vi "Test My Singleton Module API.vi"() -> ()   [LabVIEW 2017]
doc: "My Singleton Module API Tester.\n_____\nBased on Delacor QMH Project Template 3.1.0.34."
uses:
  My Singleton Module.lvlib
panel:
  out "LED":bool
  in  "Digital control":bool
  in  "Show Block Diagram":bool
  in  "X":dbl=1.0
  out "Reply Payload":dbl
  out "Reply Received?":bool
  in  "Stop Module":bool
  in  "Start Module":bool
  out "Do Something Count":i32
  in  "Test Do Something Else and Wait for Reply":bool
  in  "Hide Module Panel":bool
  in  "Show Module Panel":bool
  in  "Test Do Something Else":bool
  in  "Test Do Something":bool
  out "Status":string
  out "Module Running?":bool
  # "This VI tests the API for the Module."
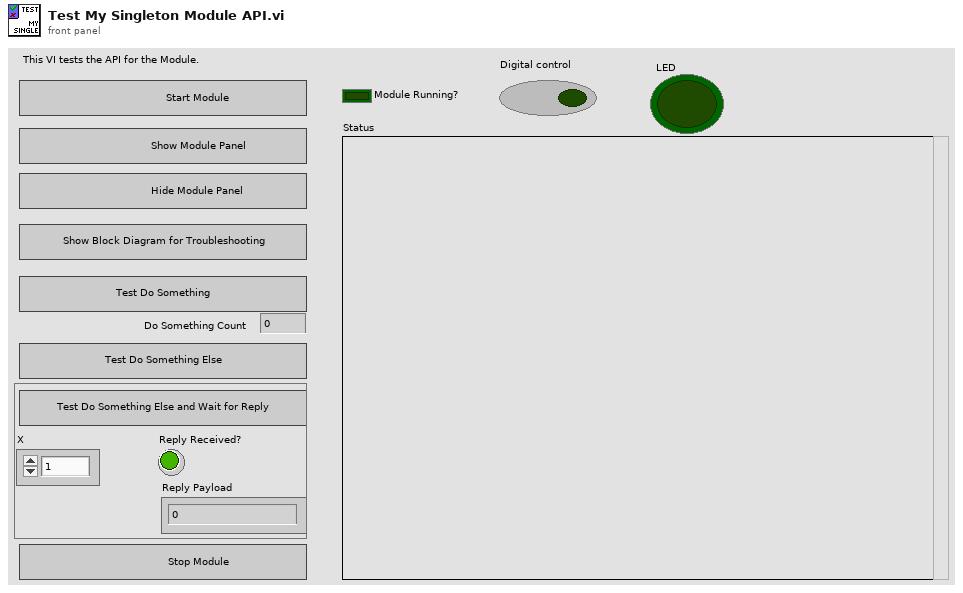
[diagram p1: front panel]
types:
  T1 = typedef "My Singleton Module.lvlib/Broadcast Events--cluster.ctl" = cluster{"Module Did Init":refnum<user-event>, "Status Updated":refnum<user-event>, "Error Reported":refnum<user-event>, "Did Something":refnum<user-event>, "Module Did Stop":refnum<user-event>, "Update Module Execution Status":refnum<user-event>}
  T2 = typedef "My Singleton Module.lvlib/Do Something Else and Wait (Reply Payload)--cluster.ctl" = cluster{"Value":dbl, "error":errorcluster}
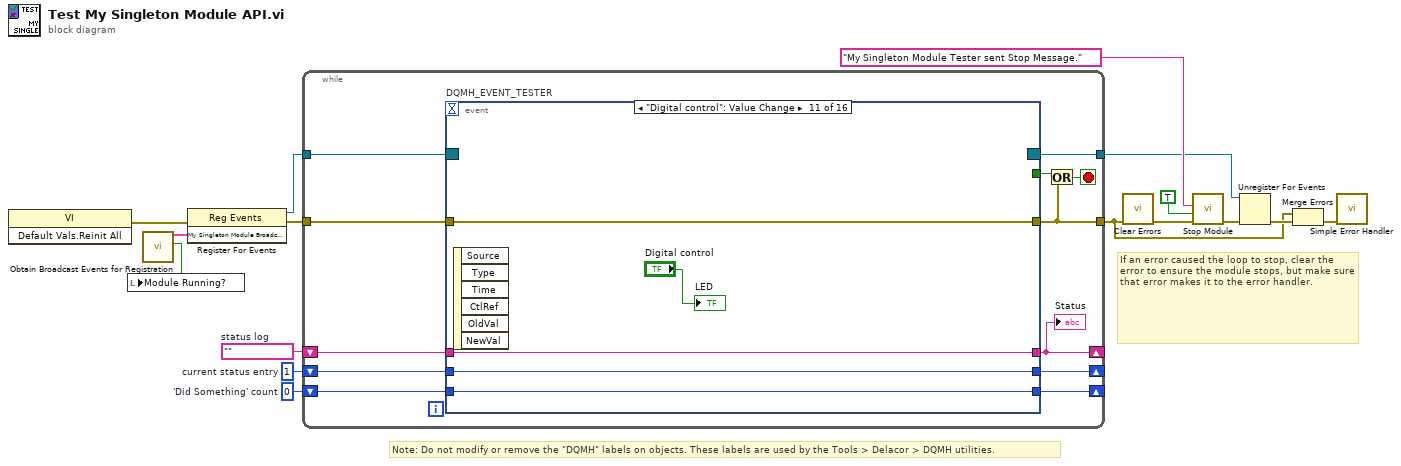
[diagram p0: block diagram]
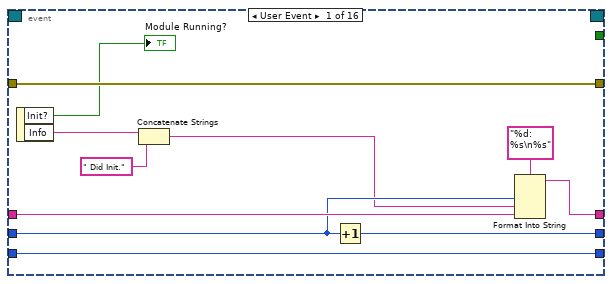
[diagram p2: hidden frame]
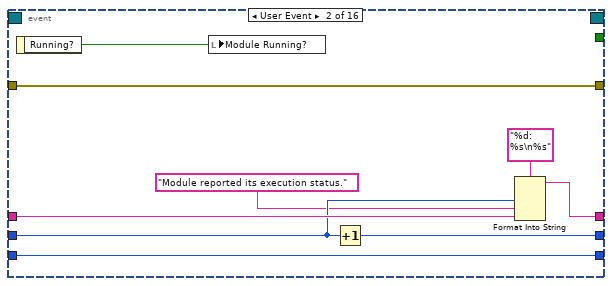
[diagram p3: hidden frame]
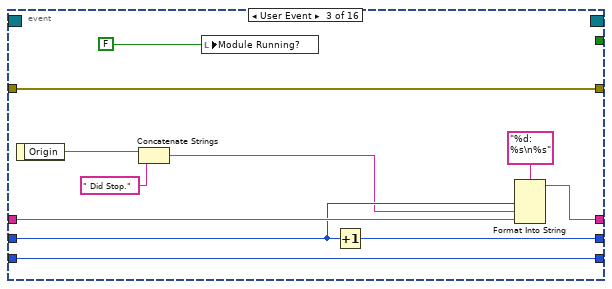
[diagram p4: hidden frame]
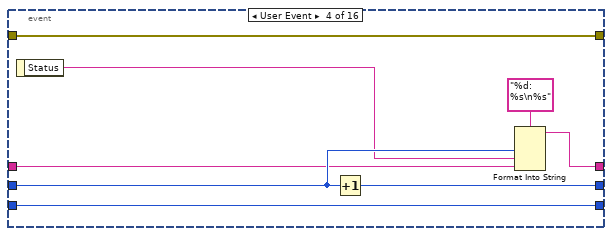
[diagram p5: hidden frame]
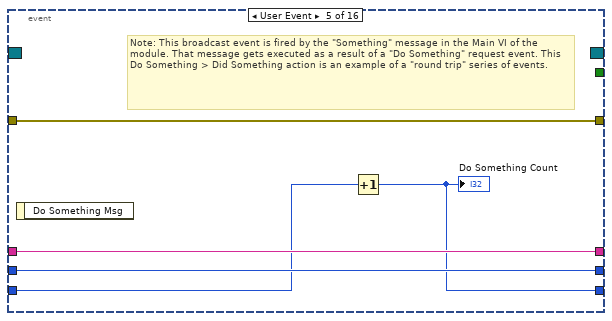
[diagram p6: hidden frame]
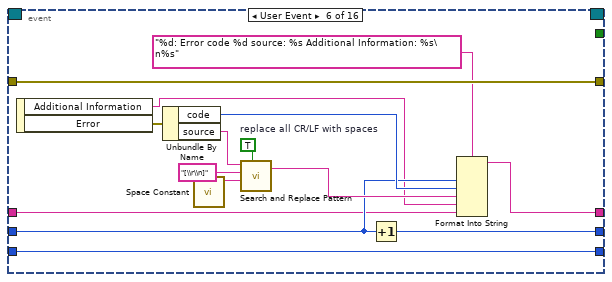
[diagram p7: hidden frame]
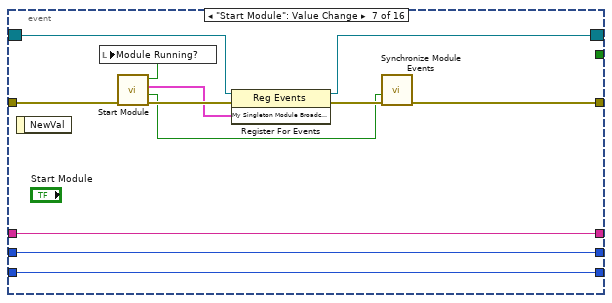
[diagram p8: hidden frame]
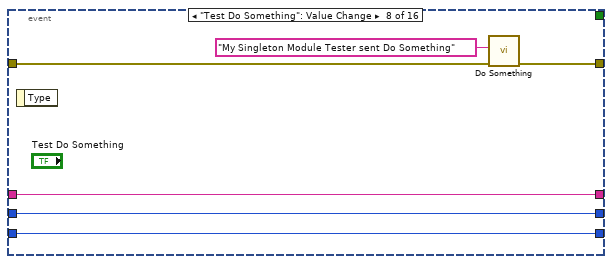
[diagram p9: hidden frame]
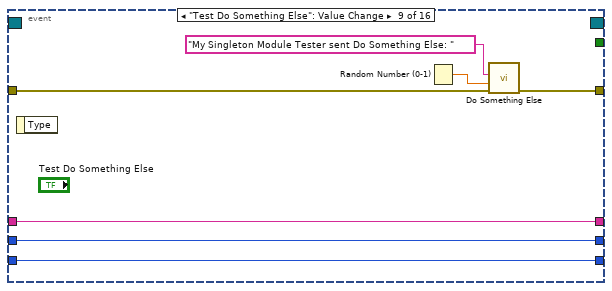
[diagram p10: hidden frame]
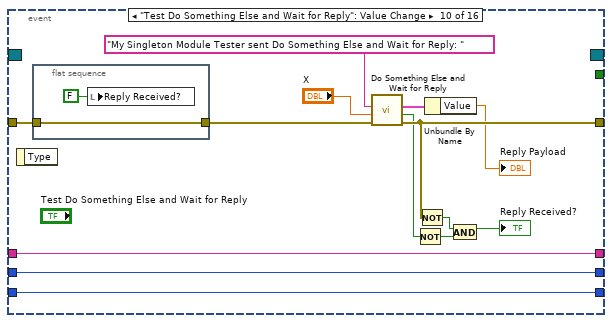
[diagram p11: hidden frame]
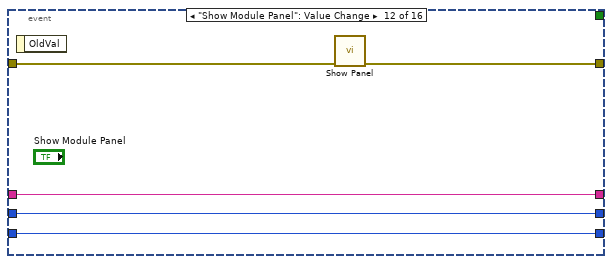
[diagram p12: hidden frame]
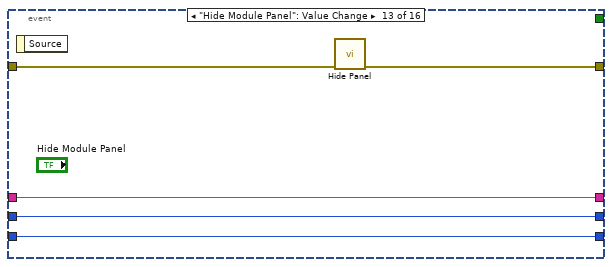
[diagram p13: hidden frame]
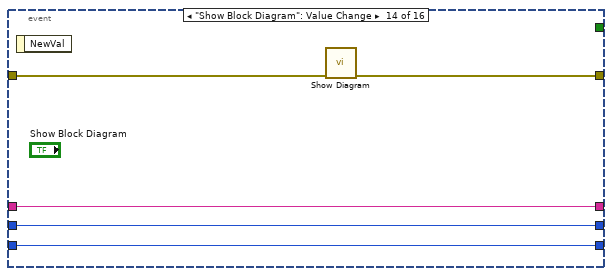
[diagram p14: hidden frame]
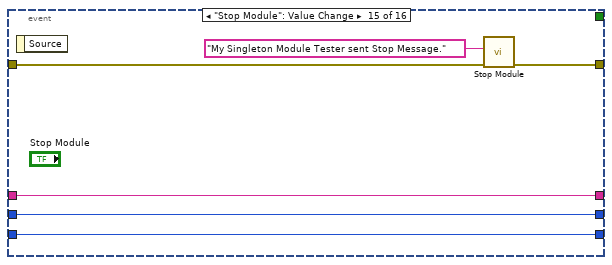
[diagram p15: hidden frame]
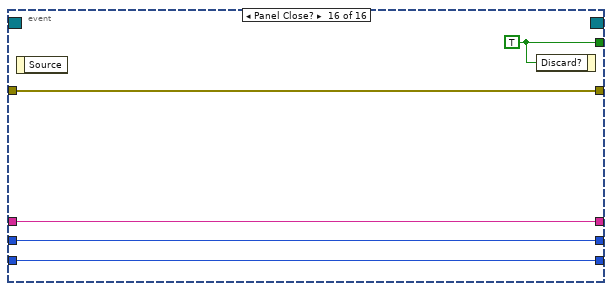
[diagram p16: hidden frame]
diagram:
  w11 = 0  # 'Did Something' count
  w12 = 1  # current status entry
  w13 = ""  # status log
  # "If an error caused the loop to stop, clear the error to ensure the module stops, but make sure that error makes it to the error handler."
  # "Note: Do not modify or remove the \"DQMH\" labels on objects. These labels are used by the Tools > Delacor > DQMH utilities."
  n1 = invoke class="VI" method="Default Vals.Reinit All"() -> (error out=w10:errorcluster)  [unwired: 3 in, 2 out]
  n2 = call "Obtain Broadcast Events for Registration.vi"() -> ("Already running?"=w1:bool, "My Singleton Module Broadcast Events"=w8:T1)  [unwired: 9 in, 1 out]
  n3 = local write "Module Running?"(w1) -> ()
  n4 = register-events(error in=w10, w8) -> (reference out=w7:refnum<event-registration>, error out=w9:errorcluster)  [unwired: 1 in]
  n5 = while {
    tunnel: w7 -> [w28]
    tunnel: [w17] -> w2
    shift-right: [w23] -> _
    shift-left: w13 -> [w25]
    shift-right: [w24] -> _
    shift-left: w12 -> [w26]
    shift-right: [w21] -> _
    shift-left: w11 -> [w22]
    tunnel: w9 -> [w19]
    tunnel: [w18] -> w6
    stop <- w20 stop-if-true
    n6 = event "DQMH_EVENT_TESTER" shown="[10] \"Digital control\": Value Change" {
      selector: w28 -> [_ _ _ _ _ _ w92 _ _ _ _ _ _ _ _ _]
      dyn-events: [_ _ _ _ _ _ w91 _ _ _ _ _ _ _ _ _] -> w18
      timeout: _ -> [_ _ _ _ _ _ _ _ _ _ _ _ _ _ _ _]
      tunnel: [_ _ _ _ _ _ _ _ _ _ _ _ _ _ _ w159] -> w27
      tunnel: [w39 w41 w49 w60 w68 w86 w90 w105 w112 w126 w133 w138 w143 w144 w151 w155] -> w17
      tunnel: w26 -> [w35 w46 w57 w64 w71 w76 w96 w102 w108 w123 w131 w136 w141 w146 w153 w157]
      tunnel: w25 -> [w36 w47 w58 w63 w72 w74 w97 w103 w109 w124 w132 w137 w142 w147 w154 w158]
      tunnel: [w33 w44 w55 w65 w72 w77 w97 w103 w109 w124 w132 w137 w142 w147 w154 w158] -> w23
      tunnel: [w34 w45 w56 w67 w71 w75 w96 w102 w108 w123 w131 w136 w141 w146 w153 w157] -> w24
      tunnel: w22 -> [w29 w42 w51 w61 w70 w87 w95 w101 w107 w122 w130 w135 w140 w145 w152 w156]
      tunnel: [w29 w42 w51 w61 w69 w87 w95 w101 w107 w122 w130 w135 w140 w145 w152 w156] -> w21
      tunnel: w19 -> [w39 w41 w49 w60 w68 w86 w89 w100 w106 w117 w133 w134 w139 w148 w149 w155]
      event User Event {
        n7 = event-data() -> ("Init?"=→"Module Running?":bool, "Info"=w32:string)  [unwired: 1 in]
        n8 = Concatenate Strings(w32, " Did Init.") -> (w31:string)
        n9 = Increment(x=w35) -> (x+1=w34:i32)
        n10 = Format Into String(format string="%d: %s\n%s", w35, w31, w36) -> (resulting string=w33:string)  [unwired: 2 in, 1 out]
      }
      event User Event {
        n11 = event-data() -> ("Running?"=w40:bool)  [unwired: 1 in]
        n12 = local write "Module Running?"(w40) -> ()
        n13 = Increment(x=w46) -> (x+1=w45:i32)
        n14 = Format Into String(format string="%d: %s\n%s", w46, "Module reported its execution status.", w47) -> (resulting string=w44:string)  [unwired: 2 in, 1 out]
      }
      event User Event {
        n15 = event-data() -> ("Origin"=w54:string)  [unwired: 1 in]
        n16 = Concatenate Strings(w54, " Did Stop.") -> (w53:string)
        n17 = local write "Module Running?"(FALSE ("Module Did Init?")) -> ()
        n18 = Increment(x=w57) -> (x+1=w56:i32)
        n19 = Format Into String(format string="%d: %s\n%s", w57, w53, w58) -> (resulting string=w55:string)  [unwired: 2 in, 1 out]
      }
      event User Event {
        n20 = event-data() -> ("Status"=w62:string)  [unwired: 1 in]
        n21 = Increment(x=w64) -> (x+1=w67:i32)
        n22 = Format Into String(format string="%d: %s\n%s", w64, w62, w63) -> (resulting string=w65:string)  [unwired: 2 in, 1 out]
      }
      event User Event {
        # "Note: This broadcast event is fired by the \"Something\" message in the Main VI of the module. That message gets executed as a result of a \"Do Something\" request event. This Do Something > Did Something action is an example of a \"round trip\" series of events."
        n23 = event-data() -> ()  [unwired: 1 in, 1 out]
        n24 = Increment(x=w70) -> (x+1=w69:i32)
        "Do Something Count" <- w69
      }
      event User Event {
        w82 = TRUE  # replace all CR/LF with spaces
        n25 = event-data() -> ("Additional Information"=w73:string, "Error"=w78:errorcluster)  [unwired: 1 in]
        n26 = Unbundle By Name(w78) -> ("code"=w79:i32, "source"=w80:string)
        n27 = call <vilib>:"Space Constant.vi"() -> ("String"=w83:string)
        n28 = call <vilib>:"Search and Replace Pattern.vi"("string"=w80, "regular expression (\"\")"="[\\r\\n]" ("regular expression (\"\")"), "replace string (\"\")"=w83, "replace all? (F)"=w82) -> ("result string"=w81:string)  [unwired: 1 in, 1 out]
        n29 = Increment(x=w76) -> (x+1=w75:i32)
        n30 = Format Into String(format string="%d: Error code %d source: %s Additional Information: %s\n%s", w76, w79, w81, w73, w74) -> (resulting string=w77:string)  [unwired: 2 in, 1 out]
      }
      event "Start Module": Value Change {
        n31 = event-data() -> ()  [unwired: 1 in, 1 out]
        n32 = call "Start Module.vi"("error in (no error)"=w89) -> ("error out"=w98:errorcluster, "Wait for Event Sync?"=w94:bool, "My Singleton Module Broadcast Events"=w93:T1, "Module Was Already Running?"=w88:bool)  [unwired: 7 in]
        n33 = local write "Module Running?"(w88) -> ()
        n34 = register-events(reference=w92, error in=w98, w93) -> (reference out=w91:refnum<event-registration>, error out=w99:errorcluster)
        n35 = call "Synchronize Module Events.vi"("error in (no error)"=w99, "Wait for Event Sync?"=w94) -> ("error out"=w90:errorcluster)  [unwired: 9 in]
      }
      event "Test Do Something": Value Change {
        n36 = event-data() -> ()  [unwired: 1 in, 1 out]
        n37 = call "Do Something.vi"("error in (no error)"=w100, "Do Something Message"="My Singleton Module Tester sent Do Something") -> ("error out"=w105:errorcluster)  [unwired: 9 in]
      }
      event "Test Do Something Else": Value Change {
        n38 = event-data() -> ()  [unwired: 1 in, 1 out]
        n39 = Random Number (0-1)() -> (number: 0 to 1=w110:dbl)
        n40 = call "Do Something Else.vi"("error in (no error)"=w106, "X"=w110, "Do Something Else Message"="My Singleton Module Tester sent Do Something Else: " ("Do Something Message")) -> ("error out"=w112:errorcluster)  [unwired: 8 in]
      }
      event "Test Do Something Else and Wait for Reply": Value Change {
        n41 = event-data() -> ()  [unwired: 1 in, 1 out]
        n42 = flat-sequence {
          tunnel: w117 -> [w128]
          tunnel: [w128] -> w116
          frame #0 {
            n43 = local write "Reply Received?"(FALSE ("Reply Received?")) -> ()
          }
        }
        n44 = call "Do Something Else and Wait for Reply.vi"("error in (no error)"=w116, "X"="X", "Do Something Else Message"="My Singleton Module Tester sent Do Something Else and Wait for Reply: " ("Do Something Message")) -> ("error out"=w126:errorcluster, "timed out?"=w121:bool, "Reply Payload"=w120:T2)  [unwired: 6 in]
        n45 = Not(x=w121) -> (.not. x?=w118:bool)
        n46 = Not(x=w126) -> (.not. x?=w113:bool)
        n47 = Unbundle By Name(w120) -> ("Value"=→"Reply Payload":dbl)
        n48 = And(x=w113, y=w118) -> (x .and. y?=→"Reply Received?":bool)
      }
      event "Digital control": Value Change {
        n49 = event-data() -> ()  [unwired: 1 in, 6 out]
        "LED" <- "Digital control"
      }
      event "Show Module Panel": Value Change {
        n50 = event-data() -> ()  [unwired: 1 in, 1 out]
        n51 = call "Show Panel.vi"("error in (no error)"=w134) -> ("error out"=w138:errorcluster)  [unwired: 10 in]
      }
      event "Hide Module Panel": Value Change {
        n52 = event-data() -> ()  [unwired: 1 in, 1 out]
        n53 = call "Hide Panel.vi"("error in (no error)"=w139) -> ("error out"=w143:errorcluster)  [unwired: 10 in]
      }
      event "Show Block Diagram": Value Change {
        n54 = event-data() -> ()  [unwired: 1 in, 1 out]
        n55 = call "Show Diagram.vi"("error in (no error)"=w148) -> ("error out"=w144:errorcluster)  [unwired: 10 in]
      }
      event "Stop Module": Value Change {
        n56 = event-data() -> ()  [unwired: 1 in, 1 out]
        n57 = call "Stop Module.vi"("error in (no error)"=w149, "Origin"="My Singleton Module Tester sent Stop Message.") -> ("error out"=w151:errorcluster)  [unwired: 9 in]
      }
      event Panel Close? {
        w159 = TRUE ("Discard?")
        n58 = event-data() -> ()  [unwired: 1 in, 1 out]
        n59 = event-data("Discard?"=w159) -> ()  [unwired: 1 in, 1 out]
      }
    }
    "Status" <- w23
    n60 = Or(x=w27, y=w17) -> (x .or. y?=w20:bool)
  }
  n61 = call <vilib>:"Clear Errors.vi"("error in (no error)"=w2) -> ("error out"=w4:errorcluster)  [unwired: 5 in, 1 out]
  n62 = call "Stop Module.vi"("error in (no error)"=w4, "Wait for Module to Stop? (F)"=TRUE ("Wait for Module to stop?"), "Origin"="My Singleton Module Tester sent Stop Message.") -> ("error out"=w15:errorcluster)  [unwired: 8 in]
  n63 = Unregister For Events(event registration refnum=w6, error in=w15) -> (error out=w16:errorcluster)
  n64 = Merge Errors(w2, w16) -> (w3:errorcluster)
  n65 = call <vilib>:"Simple Error Handler.vi"("error in (no error)"=w3) -> ()  [unwired: 4 in, 5 out]
